vi "1. Фильтр НЧ.vi"() -> ()   [LabVIEW 2020]
panel:
  in  "Stop Button":bool
  out "График демодулированного АМ-сигнала":dbl[](graph)
  out "Частота демодулированного\nсигнала, Гц":u32
  out "Коэффициент\nмодуляции":dbl
  out "График АМ-сигнала":dbl[](graph)
  in  "Амплитуда несущего\nсигнала, В":dbl(knob) scale=0.0..0.31 scale format="%#_2g"
  in  "Частота \nмодулирующего \nсигнала, Гц":u32(knob) scale=20.0..360.0
  in  "Амплитуда \nмодулирующего\nсигнала, В":dbl(knob) scale=0.0..0.31 scale format="%#_2g"
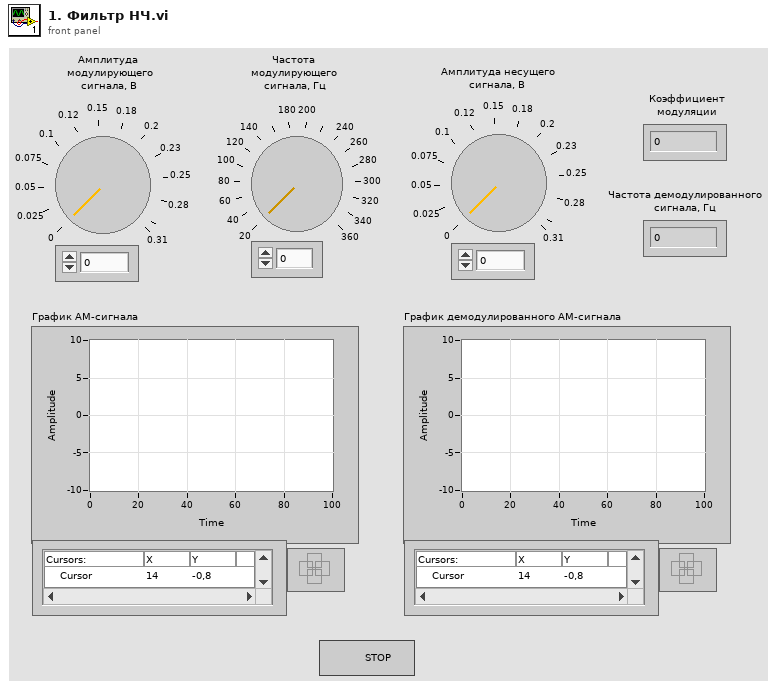
[diagram p1: front panel]
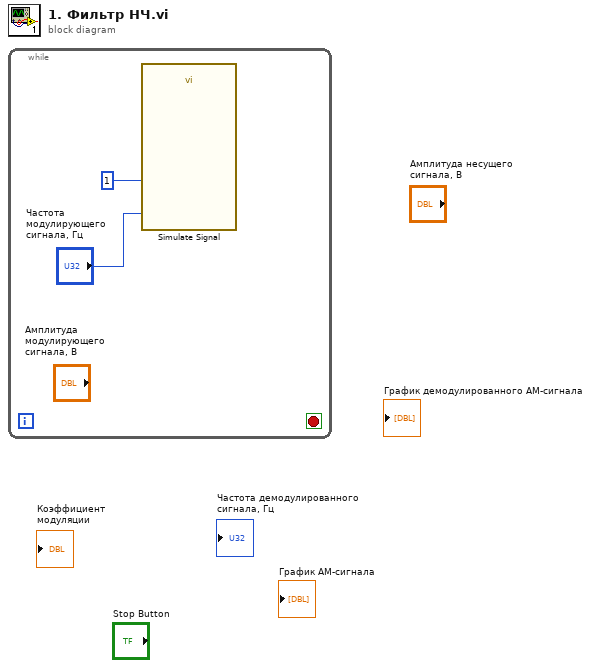
[diagram p0: block diagram]
diagram:
  n1 = while {
    stop <- _ stop-if-true
    n2 = call "Simulate Signal"("Frequency"="Частота \nмодулирующего \nсигнала, Гц", "Amplitude"=1) -> ()  [unwired: 12 in, 2 out]
  }
